vi "Chart-Check Limit.vi"(8 "error in (no error)":errorcluster, 11 "XY Graph Ref In":refnum<vi>) -> (0 "error out":errorcluster, 3 "XY Graph Ref Out":refnum<vi>)   [LabVIEW 2020]
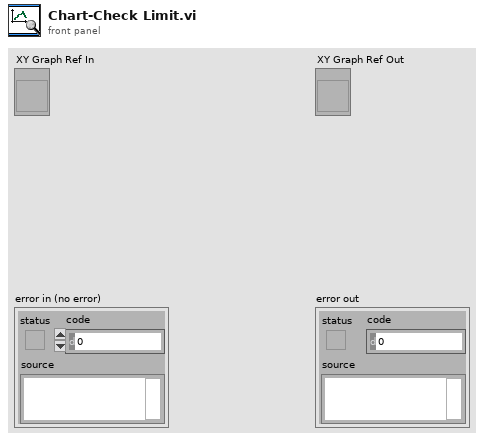
[diagram p1: front panel]
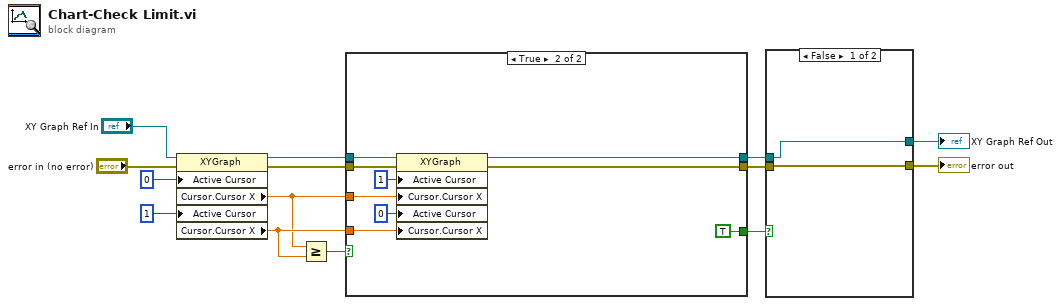
[diagram p0: block diagram]
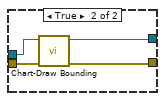
[diagram p2: hidden frame]
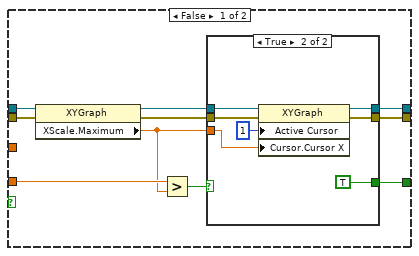
[diagram p3: hidden frame]
diagram:
  n1 = property class="XYGraph"(reference="XY Graph Ref In", error in="error in (no error)", "Active Cursor"=u32 0, "Active Cursor"=u32 1) -> (reference out=w8:refnum<vi>, error out=w9:errorcluster, "Cursor.Cursor X"=w6:dbl, "Cursor.Cursor X"=w7:dbl)
  n2 = Greater Or Equal?(x=w6, y=w7) -> (x >= y?=w10:bool)
  n3 = case shown="True" w10 {
    tunnel: w9 -> [w24 w41]
    tunnel: w8 -> [w23 w42]
    tunnel: w7 -> [w22 w39]
    tunnel: w6 -> [_ w35]
    tunnel: [w17 w37] -> w4
    tunnel: [w16 w36] -> w3
    tunnel: [w15 TRUE] -> w5
    frame False {
      n4 = property on="Property Node" class="XYGraph"(reference=w23, error in=w24) -> (reference out=w19:refnum<vi>, error out=w20:errorcluster, "XScale.Maximum"=w18:dbl)
      n5 = Greater?(x=w22, y=w18) -> (0:w21:bool)
      n6 = case shown="True" w21 {
        tunnel: w20 -> [w26 w33]
        tunnel: w19 -> [w25 w32]
        tunnel: w18 -> [_ w30]
        tunnel: [w26 w29] -> w17
        tunnel: [w25 w28] -> w16
        tunnel: [_ TRUE] -> w15
        frame False {
        }
        frame True {
          n7 = property class="XYGraph"(reference=w32, error in=w33, "Active Cursor"=u32 1, "Cursor.Cursor X"=w30) -> (reference out=w28:refnum<vi>, error out=w29:errorcluster)
        }
      }
    }
    frame True {
      n8 = property class="XYGraph"(reference=w42, error in=w41, "Active Cursor"=u32 1, "Cursor.Cursor X"=w35, "Active Cursor"=u32 0, "Cursor.Cursor X"=w39) -> (reference out=w36:refnum<vi>, error out=w37:errorcluster)
    }
  }
  n9 = case shown="False" w5 {
    tunnel: w4 -> [w44 w48]
    tunnel: w3 -> [w43 w47]
    tunnel: [w44 w46] -> w2
    tunnel: [w43 w45] -> w1
    frame False {
    }
    frame True {
      n10 = call "Chart-Draw Bounding.vi"("error in (no error)"=w48, "XY Graph Ref In"=w47) -> ("error out"=w46:errorcluster, "XY Graph Ref Out"=w45:refnum<vi>)  [unwired: 8 in]
    }
  }
  "error out" <- w2
  "XY Graph Ref Out" <- w1
